vi "Global Variable_Pixel Clock.vi"() -> ()   [LabVIEW 2015]
panel:
  out "Pixel clock_Global":bool
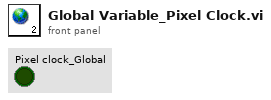
[diagram p1: front panel]
diagram:
